vi "Zstd code to error.vi"(8 "error in":errorcluster, 10 "Error code":i32, 11 "lvzstd in":refnum<class "lvzstd.lvclass">) -> (0 "error in (no error)":errorcluster, 3 "lvzstd out":refnum<class "lvzstd.lvclass">)   [LabVIEW 2020, in "lvzstd.lvlib" / "lvzstd.lvclass"]
uses:
  lvzstd.lvclass
  <vilib>/Utility/error.llb/Error Cluster From Error Code.vi
  <vilib>/ErrorRing/Error Ring.xnode
  lvzstd.lvclass/lvzstd.ctl
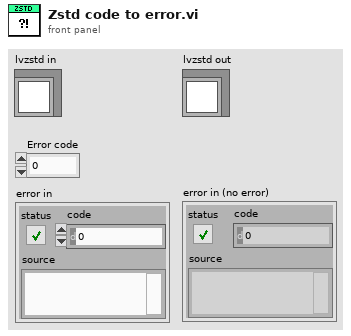
[diagram p1: front panel]
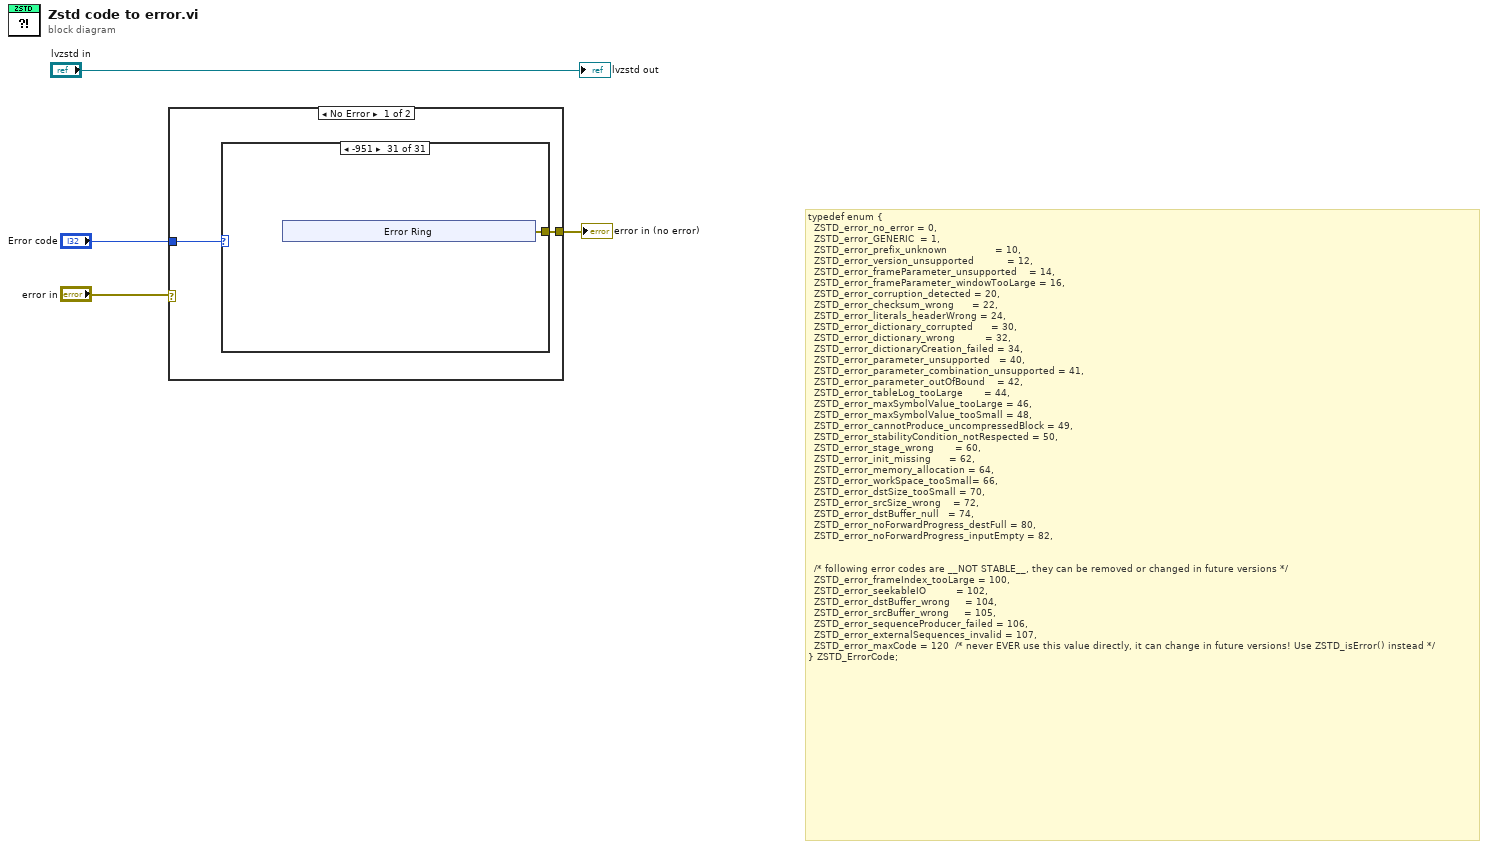
[diagram p0: block diagram]
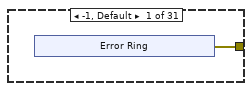
[diagram p2: hidden frame]
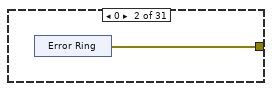
[diagram p3: hidden frame]
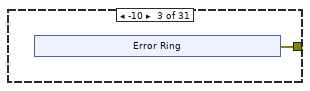
[diagram p4: hidden frame]
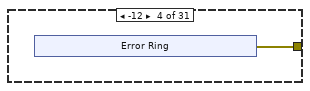
[diagram p5: hidden frame]
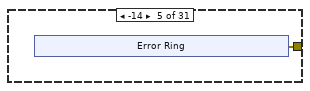
[diagram p6: hidden frame]
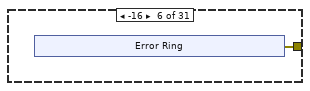
[diagram p7: hidden frame]
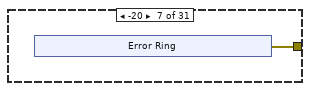
[diagram p8: hidden frame]
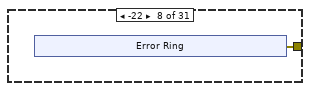
[diagram p9: hidden frame]
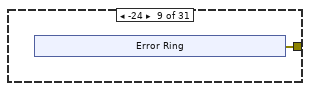
[diagram p10: hidden frame]
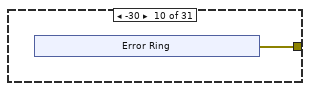
[diagram p11: hidden frame]
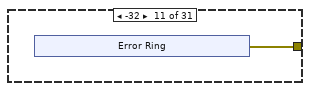
[diagram p12: hidden frame]
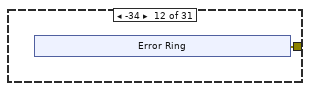
[diagram p13: hidden frame]
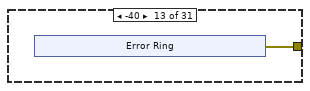
[diagram p14: hidden frame]
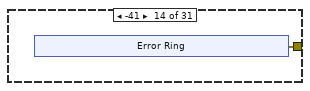
[diagram p15: hidden frame]
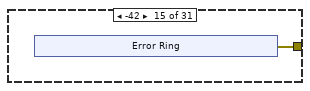
[diagram p16: hidden frame]
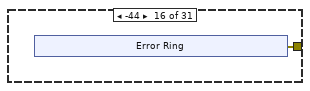
[diagram p17: hidden frame]
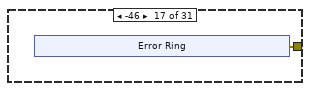
[diagram p18: hidden frame]
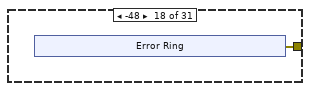
[diagram p19: hidden frame]
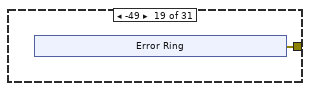
[diagram p20: hidden frame]
diagram:
  # "typedef enum {\n  ZSTD_error_no_error = 0,\n  ZSTD_error_GENERIC  = 1,\n  ZSTD_error_prefix_unknown                = 10,\n  ZSTD_error_version_unsupported           = 12,\n  ZSTD_error_frameParameter_unsupported    = 14,\n  ZSTD_error_frameParameter_windowTooLarge = 16,\n  ZSTD_error_corruption_detected = 20,\n  ZSTD_error_checksum_wrong      = 22,\n  ZSTD_error_literals_headerWrong = 24,\n  ZSTD_error_dictionary_corrupted      = 30,\n  ZSTD_error_dictionary_wrong          = 32,\n  ZSTD_error_dictionaryCreation_failed = 34,\n  ZSTD_error_parameter_unsupported   = 40,\n  ZSTD_error_parameter_combination_unsupported = 41,\n  ZSTD_error_parameter_outOfBound    = 42,\n  ZSTD_error_tableLog_tooLarge       = 44,\n  ZSTD_error_maxSymbolValue_tooLarge = 46,\n  ZSTD_error_maxSymbolValue_tooSmall = 48,\n  ZSTD_error_cannotProduce_uncompressedBlock = 49,\n  ZSTD_error_stabilityCondition_notRespected = 50,\n  ZSTD_error_stage_wrong       = 60,\n  ZSTD_error_init_missing      = 62,\n  ZSTD_error_memory_allocation = 64,\n  ZSTD_error_workSpace_tooSmall= 66,\n  ZSTD_error_dstSize_tooSmall = 70,\n  ZSTD_error_srcSize_wrong    = 72,\n  ZSTD_error_dstBuffer_null   = 74,\n  ZSTD_error_noForwardProgress_destFull = 80,\n  ZSTD_error_noForwardProgress_inputEmpty = 82,\n\n\n  /* following error codes are __NOT STABLE__, they can be removed or changed in future versions */\n  ZSTD_error_frameIndex_tooLarge = 100,\n  ZSTD_error_seekableIO          = 102,\n  ZSTD_error_dstBuffer_wrong     = 104,\n  ZSTD_error_srcBuffer_wrong     = 105,\n  ZSTD_error_sequenceProducer_failed = 106,\n  ZSTD_error_externalSequences_invalid = 107,\n  ZSTD_error_maxCode = 120  /* never EVER use this value directly, it can change in future versions! Use ZSTD_isError() instead */\n} ZSTD_ErrorCode;"
  n1 = case shown="No Error" "error in" {
    selector: "error in" -> [_ w159]
    tunnel: "Error code" -> [w6 _]
    tunnel: [w5 w159] -> w3
    frame No Error {
      n2 = case shown="-951" w6 {
        tunnel: [w7 w12 w14 w19 w24 w29 w34 w39 w44 w49 w54 w59 w64 w69 w74 w79 w84 w89 w94 w99 w104 w109 w114 w119 w124 w129 w134 w139 w144 w149 w154] -> w5
        frame -1, Default {
          n3 = xnode "Error Ring"() -> ("error out"=w7:errorcluster)
        }
        frame 0 {
          n4 = xnode "Error Ring"() -> ("error out"=w12:errorcluster)
        }
        frame -10 {
          n5 = xnode "Error Ring"() -> ("error out"=w14:errorcluster)
        }
        frame -12 {
          n6 = xnode "Error Ring"() -> ("error out"=w19:errorcluster)
        }
        frame -14 {
          n7 = xnode "Error Ring"() -> ("error out"=w24:errorcluster)
        }
        frame -16 {
          n8 = xnode "Error Ring"() -> ("error out"=w29:errorcluster)
        }
        frame -20 {
          n9 = xnode "Error Ring"() -> ("error out"=w34:errorcluster)
        }
        frame -22 {
          n10 = xnode "Error Ring"() -> ("error out"=w39:errorcluster)
        }
        frame -24 {
          n11 = xnode "Error Ring"() -> ("error out"=w44:errorcluster)
        }
        frame -30 {
          n12 = xnode "Error Ring"() -> ("error out"=w49:errorcluster)
        }
        frame -32 {
          n13 = xnode "Error Ring"() -> ("error out"=w54:errorcluster)
        }
        frame -34 {
          n14 = xnode "Error Ring"() -> ("error out"=w59:errorcluster)
        }
        frame -40 {
          n15 = xnode "Error Ring"() -> ("error out"=w64:errorcluster)
        }
        frame -41 {
          n16 = xnode "Error Ring"() -> ("error out"=w69:errorcluster)
        }
        frame -42 {
          n17 = xnode "Error Ring"() -> ("error out"=w74:errorcluster)
        }
        frame -44 {
          n18 = xnode "Error Ring"() -> ("error out"=w79:errorcluster)
        }
        frame -46 {
          n19 = xnode "Error Ring"() -> ("error out"=w84:errorcluster)
        }
        frame -48 {
          n20 = xnode "Error Ring"() -> ("error out"=w89:errorcluster)
        }
        frame -49 {
          n21 = xnode "Error Ring"() -> ("error out"=w94:errorcluster)
        }
        frame -50 {
          n22 = xnode "Error Ring"() -> ("error out"=w99:errorcluster)
        }
        frame -60 {
          n23 = xnode "Error Ring"() -> ("error out"=w104:errorcluster)
        }
        frame -62 {
          n24 = xnode "Error Ring"() -> ("error out"=w109:errorcluster)
        }
        frame -64 {
          n25 = xnode "Error Ring"() -> ("error out"=w114:errorcluster)
        }
        frame -66 {
          n26 = xnode "Error Ring"() -> ("error out"=w119:errorcluster)
        }
        frame -70 {
          n27 = xnode "Error Ring"() -> ("error out"=w124:errorcluster)
        }
        frame -72 {
          n28 = xnode "Error Ring"() -> ("error out"=w129:errorcluster)
        }
        frame -74 {
          n29 = xnode "Error Ring"() -> ("error out"=w134:errorcluster)
        }
        frame -80 {
          n30 = xnode "Error Ring"() -> ("error out"=w139:errorcluster)
        }
        frame -82 {
          n31 = xnode "Error Ring"() -> ("error out"=w144:errorcluster)
        }
        frame -950 {
          n32 = xnode "Error Ring"() -> ("error out"=w149:errorcluster)
        }
        frame -951 {
          n33 = xnode "Error Ring"() -> ("error out"=w154:errorcluster)
        }
      }
    }
    frame Error {
    }
  }
  "error in (no error)" <- w3
  "lvzstd out" <- "lvzstd in"
